vi "AMZ_S3_APIHLP_Parse Complete Multipart Upload Result.vi"(8 "error in (no error)":errorcluster, 10 "Response body":string, 11 "Response header":string) -> (0 "error out":errorcluster, 2 "Version ID":string, 3 "CompleteMultipartUploadResult":T1)   [LabVIEW 2015, in "LV Interface for Amazon S3.lvlib"]
uses:
  LV Interface for Amazon S3.lvlib
  Typedefs/AMZ_S3_API_CompleteMultipartUploadResult.ctl
  XML Parser/XML Parser.lvlib
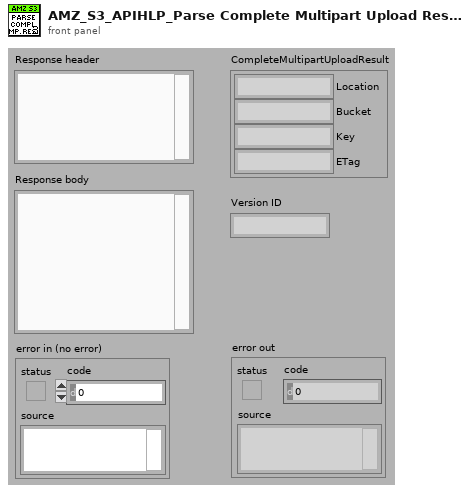
[diagram p1: front panel]
types:
  T1 = typedef "LV Interface for Amazon S3.lvlib/AMZ_S3_API_CompleteMultipartUploadResult.ctl" = cluster{"Location":string, "Bucket":string, "Key":string, "ETag":string}
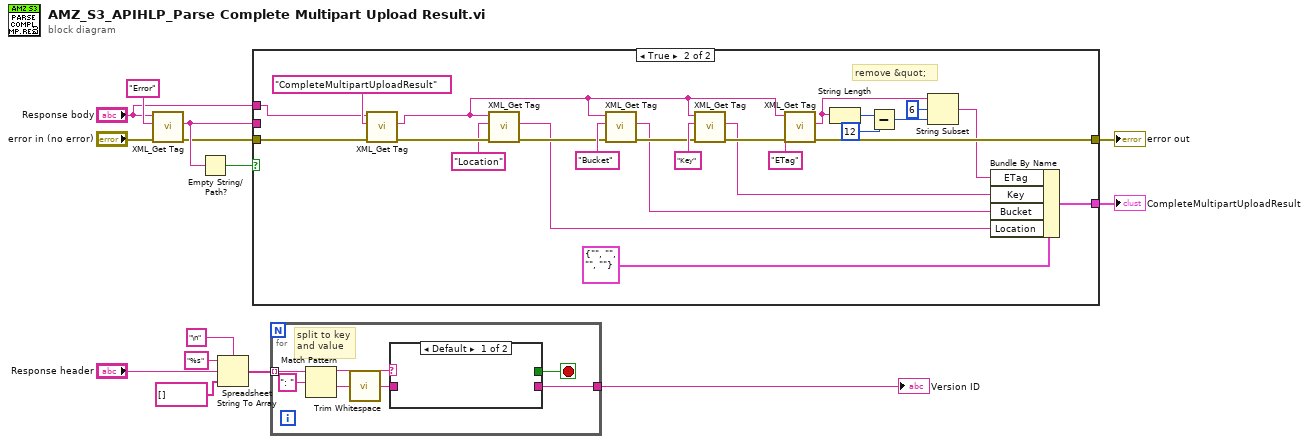
[diagram p0: block diagram]
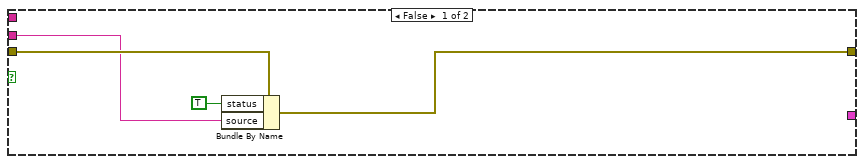
[diagram p2: hidden frame]
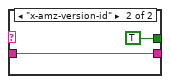
[diagram p3: hidden frame]
diagram:
  n1 = call "XML_Get Tag.vi"("error in (no error)"="error in (no error)", "Tag name"="Error", "XML String in"="Response body") -> ("error out"=w1:errorcluster, "Tag value"=w2:string)  [unwired: 4 in, 3 out]
  n2 = Empty String/Path?(string/path=w2) -> (empty?=w4:bool)
  n3 = Spreadsheet String To Array(delimiter (Tab)="\n", format string="%s", spreadsheet string="Response header", array type (2D Dbl)=string[] []) -> (array=w10:string[])
  n4 = case shown="True" w4 {
    tunnel: [w15 w33] -> w14
    tunnel: [_ w32] -> w13
    tunnel: "Response body" -> [_ w19]
    tunnel: w2 -> [w16 _]
    tunnel: w1 -> [w18 w20]
    frame False {
      n5 = Bundle By Name(cluster=w18, "status"=TRUE, "source"=w16) -> (w15:errorcluster)
    }
    frame True {
      # "remove &quot;"
      n6 = call "XML_Get Tag.vi"("error in (no error)"=w20, "Tag name"="CompleteMultipartUploadResult", "XML String in"=w19) -> ("error out"=w31:errorcluster, "Tag value"=w30:string)  [unwired: 4 in, 3 out]
      n7 = call "XML_Get Tag.vi"("error in (no error)"=w31, "Tag name"="Location", "XML String in"=w30) -> ("error out"=w28:errorcluster, "Tag value"=w27:string)  [unwired: 4 in, 3 out]
      n8 = call "XML_Get Tag.vi"("error in (no error)"=w28, "Tag name"="Bucket", "XML String in"=w30) -> ("error out"=w39:errorcluster, "Tag value"=w35:string)  [unwired: 4 in, 3 out]
      n9 = call "XML_Get Tag.vi"("error in (no error)"=w39, "Tag name"="Key", "XML String in"=w30) -> ("error out"=w37:errorcluster, "Tag value"=w34:string)  [unwired: 4 in, 3 out]
      n10 = call "XML_Get Tag.vi"("error in (no error)"=w37, "Tag name"="ETag", "XML String in"=w30) -> ("error out"=w33:errorcluster, "Tag value"=w25:string)  [unwired: 4 in, 3 out]
      n11 = String Length(string=w25) -> (length=w24:i32)
      n12 = Subtract(x=w24, y=12) -> (x-y=w22:i32)
      n13 = String Subset(string=w25, offset (0)=6, length (rest)=w22) -> (substring=w21:string)
      n14 = Bundle By Name(cluster=T1 {"Location"="", "Bucket"="", "Key"="", "ETag"=""} ("CompleteMultipartUploadResult"), "ETag"=w21, "Key"=w34, "Bucket"=w35, "Location"=w27) -> (w32:T1)
    }
  }
  "CompleteMultipartUploadResult" <- w13
  "error out" <- w14
  n15 = for {
    tunnel: w10 -> [w49] mode=indexing
    tunnel: [w43] -> w8
    stop <- w44 stop-if-true
    # "split to key\nand value"
    n16 = Match Pattern(string=w49, regular expression=": ") -> (before substring=w47:string, after substring=w46:string)  [unwired: 1 in, 2 out]
    n17 = call <vilib>:"Trim Whitespace.vi"("string"=w46) -> ("trimmed string"=w45:string)  [unwired: 1 in]
    n18 = case shown="Default" w47 {
      tunnel: w45 -> [_ w51]
      tunnel: [_ w51] -> w43
      tunnel: [_ TRUE] -> w44
      frame Default {
      }
      frame "x-amz-version-id" {
      }
    }
  }
  "Version ID" <- w8
